vi "LJM logger append to array if smaller than default.vi"(2 "Default Bool Array":bool[](array[boolean]), 3 "Bool Array to Check":bool[](array[boolean]), 4 "Default String Array":string[](array[string]), 5 "String Array to Check":string[](array[string])) -> (0 "Output Bool Array":bool[](array[boolean]), 1 "Output String Array":string[](array[string]))   [LabVIEW 2026]
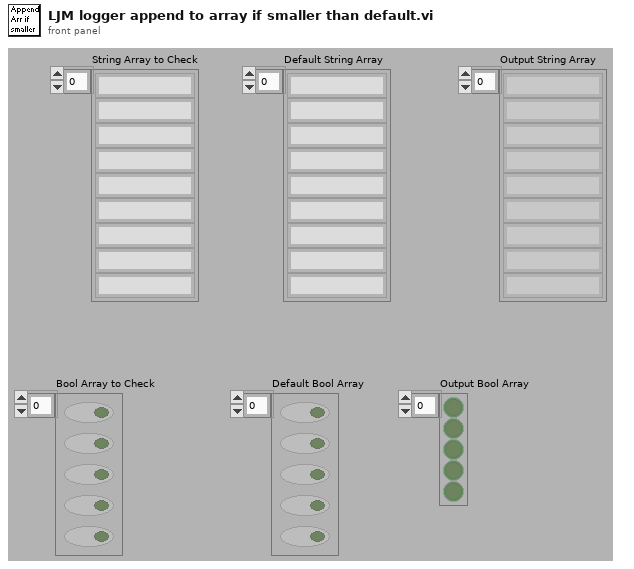
[diagram p1: front panel]
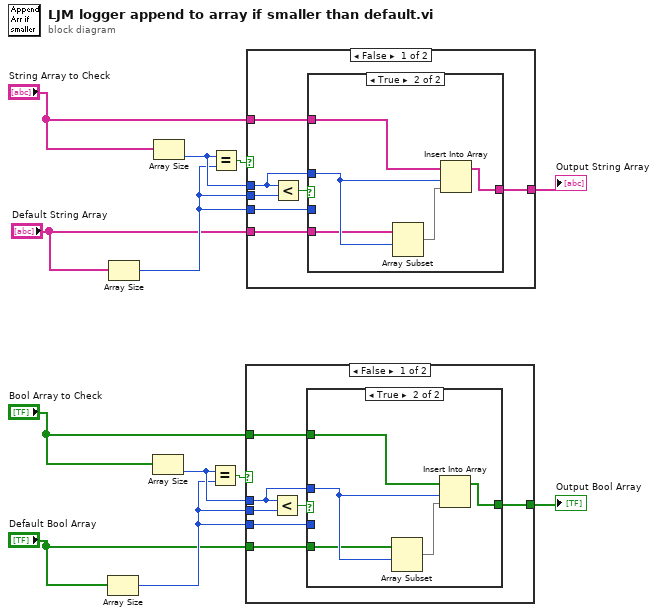
[diagram p0: block diagram]
diagram:
  n1 = Array Size(array="Default Bool Array") -> (size(s)=w4:i32)
  n2 = Array Size(array="Default String Array") -> (size(s)=w10:i32)
  n3 = Array Size(array="Bool Array to Check") -> (size(s)=w5:i32)
  n4 = Array Size(array="String Array to Check") -> (size(s)=w11:i32)
  n5 = Equal?(x=w5, y=w4) -> (x = y?=w6:bool)
  n6 = Equal?(x=w11, y=w10) -> (x = y?=w12:bool)
  n7 = case shown="False" w6 {
    tunnel: w5 -> [w14 _]
    tunnel: w4 -> [w19 _]
    tunnel: w4 -> [w17 _]
    tunnel: "Bool Array to Check" -> [w16 w26]
    tunnel: [w15 w26] -> w1
    tunnel: "Default Bool Array" -> [w13 _]
    frame False {
      n8 = Less?(x=w14, y=w19) -> (x < y?=w18:bool)
      n9 = case shown="True" w18 {
        tunnel: w17 -> [_ _]
        tunnel: w16 -> [w20 w25]
        tunnel: [w20 w21] -> w15
        tunnel: w14 -> [_ w24]
        tunnel: w13 -> [_ w23]
        frame False {
        }
        frame True {
          n10 = Array Subset(array=w23, index=w24) -> (w22:bool[])  [unwired: 1 in]
          n11 = Insert Into Array(array=w25, index=w24, new element=w22) -> (w21:bool[])
        }
      }
    }
    frame True {
    }
  }
  "Output Bool Array" <- w1
  n12 = case shown="False" w12 {
    tunnel: w11 -> [w28 _]
    tunnel: w10 -> [w33 _]
    tunnel: w10 -> [w31 _]
    tunnel: "String Array to Check" -> [w30 w40]
    tunnel: [w29 w40] -> w7
    tunnel: "Default String Array" -> [w27 _]
    frame False {
      n13 = Less?(x=w28, y=w33) -> (x < y?=w32:bool)
      n14 = case shown="True" w32 {
        tunnel: w31 -> [_ _]
        tunnel: w30 -> [w34 w39]
        tunnel: [w34 w35] -> w29
        tunnel: w28 -> [_ w38]
        tunnel: w27 -> [_ w37]
        frame False {
        }
        frame True {
          n15 = Array Subset(array=w37, index=w38) -> (w36:string[])  [unwired: 1 in]
          n16 = Insert Into Array(array=w39, index=w38, new element=w36) -> (w35:string[])
        }
      }
    }
    frame True {
    }
  }
  "Output String Array" <- w7
